vi "__uintDividetest.vi"(3 "Base (decimal)":T1=10 items=["Binary"=2, "Octal"=8, "Decimal"=10, "Hexadecimal"=16, "Hexatrigesimal"=36], 4 "Uint2 in":u8[](array[numeric]), 5 "Uint1 in":u8[](array[numeric])) -> (0 "Timing division":u32, 1 "floor(Uint1 / Uint1)":u8[](array[numeric]), 2 "Uint1 - Uint2 * floor(Uint1 / Uint2)":u8[](array[numeric]))   [LabVIEW 2011]
uses:
  enumBase.ctl
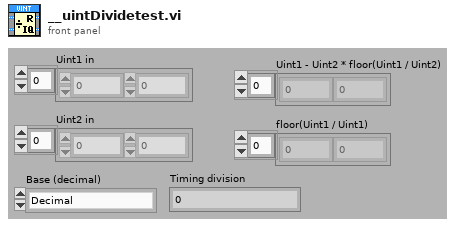
[diagram p1: front panel]
types:
  T1 = typedef "enumBase.ctl" = u16
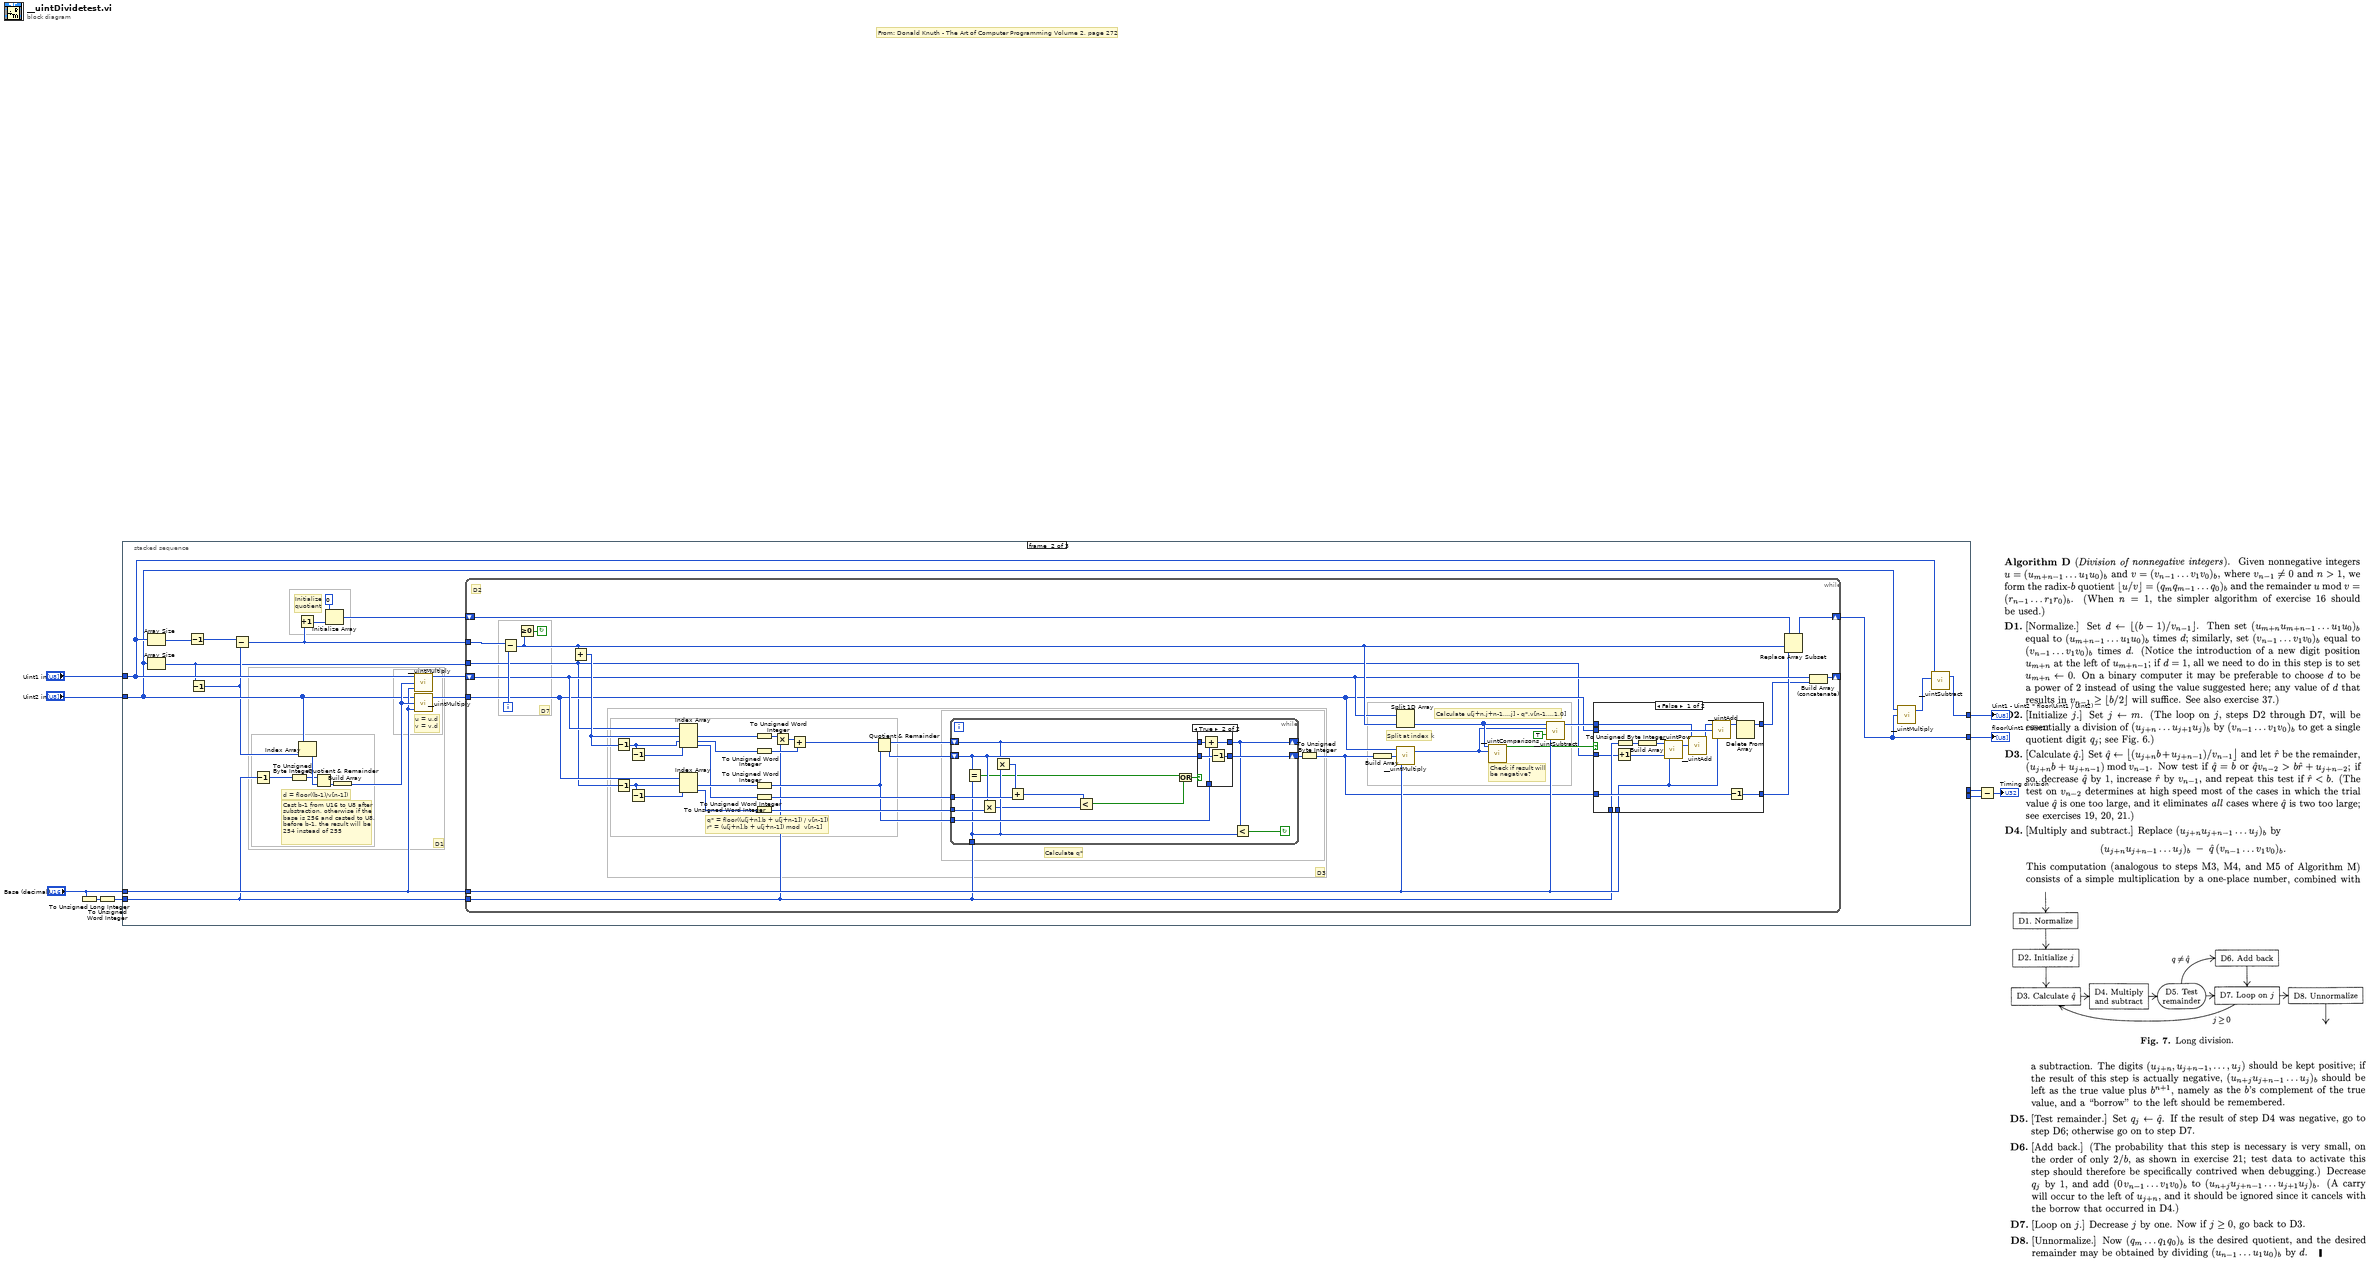
[diagram p0: block diagram]
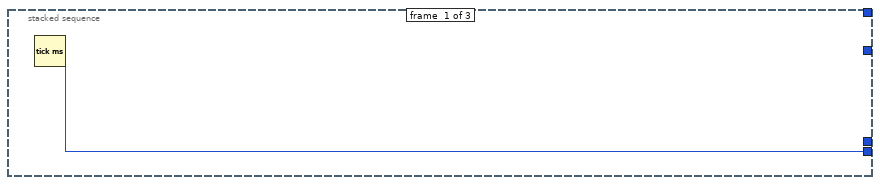
[diagram p2: hidden frame]
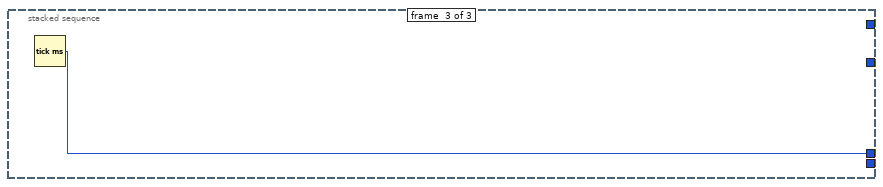
[diagram p5: hidden frame]
diagram:
  # "From: Donald Knuth - The Art of Computer Programming Volume 2, page 272"
  n1 = To Unsigned Long Integer(number="Base (decimal)") -> (unsigned 32bit integer=w1:u32)
  n2 = To Unsigned Word Integer(number=w1) -> (unsigned 16bit integer=w3:u16)
  n3 = stacked-sequence {
    tunnel: "Uint2 in" -> [_ w20 _]
    tunnel: "Uint1 in" -> [_ w23 _]
    tunnel: [w11 _ _] -> w9
    tunnel: [_ _ w113] -> w8
    tunnel: "Base (decimal)" -> [_ w26 _]
    tunnel: [_ w22 _] -> w5
    tunnel: [_ w19 _] -> w4
    tunnel: w3 -> [_ w15 _]
    frame #0 {
      n4 = Tick Count (ms)() -> (millisecond timer value=w11:u32)
    }
    frame #1 {
      # "D1"
      # "Cast b-1 from U16 to U8 after\nsubstraction, otherwise if the\nbase is 256 and casted to U8,\nbefore b-1, the result will be\n254 instead of 255"
      # "Initialize\nquotient"
      # "u = u.d \nv = v.d"
      # "d = floor((b-1)/v[n-1])"
      n5 = Array Size(array=w23) -> (size(s)=w29:i32)
      n6 = Array Size(array=w20) -> (size(s)=w14:i32)
      n7 = Decrement(x=w29) -> (x-1=w18:i32)
      n8 = Decrement(x=w14) -> (x-1=w17:i32)
      n9 = Subtract(x=w18, y=w17) -> (x-y=w13:i32)
      n10 = Decrement(x=w15) -> (x-1=w33:u16)
      n11 = To Unsigned Byte Integer(number=w33) -> (unsigned 8bit integer=w16:u8)
      n12 = Increment(x=w13) -> (x+1=w12:i32)
      n13 = Index Array(array=w20, index=w17) -> (element=w32:u8)
      n14 = Quotient & Remainder(x=w16, y=w32) -> (floor(x/y)=w31:u8)  [unwired: 1 out]
      n15 = Initialize Array(u8 0, w12) -> (w24:u8[])
      n16 = Build Array(w31) -> (w30:u8[])
      n17 = call "__uintMultiply.vi"("Base (decimal)"=w26, "UInt2 in"=w30, "UInt1 in"=w23) -> ("UInt1 * Uint2"=w28:u8[])  [unwired: 1 out]
      n18 = call "__uintMultiply.vi"("Base (decimal)"=w26, "UInt2 in"=w30, "UInt1 in"=w20) -> ("UInt1 * Uint2"=w27:u8[])  [unwired: 1 out]
      n19 = while {
        tunnel: w13 -> [w50]
        tunnel: w14 -> [w34]
        tunnel: w27 -> [w36]
        tunnel: w15 -> [w35]
        tunnel: w26 -> [w51]
        shift-right: [w46] -> w22
        shift-left: w24 -> [w45]
        shift-right: [w43] -> _
        shift-left: w28 -> [w44]
        i -> [w49]
        stop <- w47 continue-if-true
        # "D2"
        # "Calculate u[j+n,j+n-1,..,j] - q*.v[n-1,..,1,0]"
        # "D3"
        # "D7"
        # "Check if result will\nbe negative?"
        # "Split at index k"
        # "Calculate q*"
        # "q* = floor((u[j+n].b + u[j+n-1]) / v[n-1])\nr* = (u[j+n].b + u[j+n-1]) mod  v[n-1]"
        n20 = Subtract(x=w50, y=w49) -> (x-y=w48:i32)
        n21 = Greater Or Equal To 0?(x=w48) -> (x >= 0?=w47:bool)
        n22 = Add(x=w48, y=w34) -> (x+y=w72:i32)
        n23 = Decrement(x=w72) -> (x-1=w61:i32)
        n24 = Decrement(x=w34) -> (x-1=w66:i32)
        n25 = Decrement(x=w61) -> (x-1=w62:i32)
        n26 = Decrement(x=w66) -> (x-1=w65:i32)
        n27 = Index Array(array=w44, index #1=w72, index #2=w61, index #3=w62) -> (element #1=w74:u8, element #2=w70:u8, element #3=w60:u8)
        n28 = Index Array(array=w36, index #1=w66, index #2=w65) -> (element #1=w67:u8, element #2=w64:u8)
        n29 = To Unsigned Word Integer(number=w74) -> (unsigned 16bit integer=w73:u16)
        n30 = To Unsigned Word Integer(number=w70) -> (unsigned 16bit integer=w69:u16)
        n31 = To Unsigned Word Integer(number=w67) -> (unsigned 16bit integer=w56:u16)
        n32 = To Unsigned Word Integer(number=w60) -> (unsigned 16bit integer=w59:u16)
        n33 = To Unsigned Word Integer(number=w64) -> (unsigned 16bit integer=w63:u16)
        n34 = Multiply(x=w73, y=w35) -> (x*y=w71:u16)
        n35 = Add(x=w71, y=w69) -> (x+y=w68:u16)
        n36 = Quotient & Remainder(x=w68, y=w56) -> (x-y*floor(x/y)=w58:u16, floor(x/y)=w57:u16)
        n37 = while {
          tunnel: w63 -> [w105]
          tunnel: w35 -> [w100]
          tunnel: w59 -> [w103]
          tunnel: w56 -> [w101]
          shift-right: [w92] -> _
          shift-left: w58 -> [w98]
          shift-right: [w99] -> w54
          shift-left: w57 -> [w102]
          stop <- w91 continue-if-true
          n38 = Equal?(x=w102, y=w100) -> (x = y?=w96:bool)
          n39 = Multiply(x=w102, y=w105) -> (x*y=w94:u16)
          n40 = Multiply(x=w98, y=w100) -> (x*y=w104:u16)
          n41 = Add(x=w104, y=w103) -> (x+y=w95:u16)
          n42 = Less?(x=w95, y=w94) -> (x < y?=w93:bool)
          n43 = Or(x=w96, y=w93) -> (x .or. y?=w97:bool)
          n44 = case shown="True" w97 {
            tunnel: w98 -> [w107 w111]
            tunnel: w102 -> [w106 w112]
            tunnel: w101 -> [_ w110]
            tunnel: [w107 w108] -> w92
            tunnel: [w106 w109] -> w99
            frame False {
            }
            frame True {
              n45 = Add(x=w111, y=w110) -> (x+y=w108:u16)
              n46 = Decrement(x=w112) -> (x-1=w109:u16)
            }
          }
          n47 = Less?(x=w92, y=w100) -> (x < y?=w91:bool)
        }
        n48 = To Unsigned Byte Integer(number=w54) -> (unsigned 8bit integer=w39:u8)
        n49 = Build Array(w39) -> (w55:u8[])
        n50 = Split 1D Array(array=w44, index=w48) -> (second subarray=w42:u8[])  [unwired: 1 out]
        n51 = call "__uintMultiply.vi"("Base (decimal)"=w51, "UInt2 in"=w55, "UInt1 in"=w36) -> ("UInt1 * Uint2"=w41:u8[])  [unwired: 1 out]
        n52 = call "__uintComparisons.vi"("Uint2 in"=w41, "Uint1 in"=w42) -> ("Uint1 >= Uint2"=w40:bool)  [unwired: 3 in, 6 out]
        n53 = call "__uintSubtract.vi"("Base (decimal)"=w51, "Difference (false)"=TRUE, "Uint2 in"=w41, "Uint1 in"=w42) -> ("Uint1 - Uint2"=w52:u8[])  [unwired: 1 out]
        n54 = case shown="False" w40 {
          tunnel: w52 -> [w83 w90]
          tunnel: [w84 w90] -> w37
          tunnel: w51 -> [w77 _]
          tunnel: w39 -> [w88 w89]
          tunnel: [w87 w89] -> w38
          tunnel: w36 -> [w85 _]
          tunnel: w35 -> [w79 _]
          tunnel: w34 -> [w76 _]
          frame False {
            n55 = Increment(x=w76) -> (x+1=w75:i32)
            n56 = To Unsigned Byte Integer(number=w79) -> (unsigned 8bit integer=w78:u8)
            n57 = Build Array(w78) -> (w80:u8[])
            n58 = call "__uintPow.vi"("Base (decimal)"=w77, "y (2)"=w75, "UInt in"=w80) -> ("UInt^y"=w81:u8[])  [unwired: 1 out]
            n59 = call "__uintAdd.vi"("Uint2 in"=w81, "Uint1 in"=w83) -> ("Uint1 + Uint2"=w82:u8[])  [unwired: 1 in, 1 out]
            n60 = call "__uintAdd.vi"("Base (decimal)"=w77, "Uint2 in"=w85, "Uint1 in"=w82) -> ("Uint1 + Uint2"=w86:u8[])  [unwired: 1 out]
            n61 = Decrement(x=w88) -> (x-1=w87:u8)
            n62 = Delete From Array(array=w86) -> (array with subset deleted=w84:u8[])  [unwired: 2 in, 1 out]
          }
          frame True {
          }
        }
        n63 = Replace Array Subset(array=w45, new element=w38, index=w48) -> (w46:u8[])
        n64 = Build Array (concatenate)(w44, w37) -> (w43:u8[])
      }
      n65 = call "__uintMultiply.vi"("UInt2 in"=w22, "UInt1 in"=w20) -> ("UInt1 * Uint2"=w21:u8[])  [unwired: 1 in, 1 out]
      n66 = call "__uintSubtract.vi"("Uint2 in"=w21, "Uint1 in"=w23) -> ("Uint1 - Uint2"=w19:u8[])  [unwired: 2 in, 1 out]
    }
    frame #2 {
      n67 = Tick Count (ms)() -> (millisecond timer value=w113:u32)
    }
  }
  "Uint1 - Uint2 * floor(Uint1 / Uint2)" <- w4
  "floor(Uint1 / Uint1)" <- w5
  n68 = Subtract(x=w8, y=w9) -> (x-y=→"Timing division":u32)
